vi "subSave_Dcimg2Bin.vi"(5 "Delete .dcimg? (T)":bool=TRUE, 7 "Text":string, 8 "Error in":errorcluster, 11 ".dcimg file name":path) -> (0 "Error out":errorcluster)   [LabVIEW 2015]
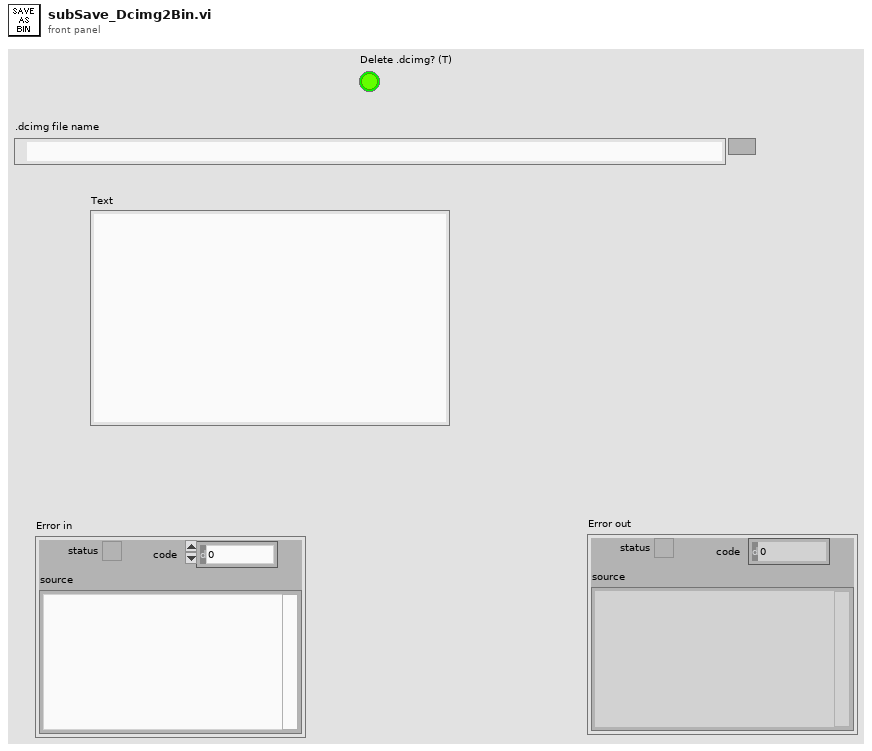
[diagram p1: front panel]
types:
  T1 = enum16{"open", "replace", "create", "open or create", "replace or create", "replace or create with confirmation"}
  T2 = enum16{"big-endian, network order", "native, host order", "little-endian"}
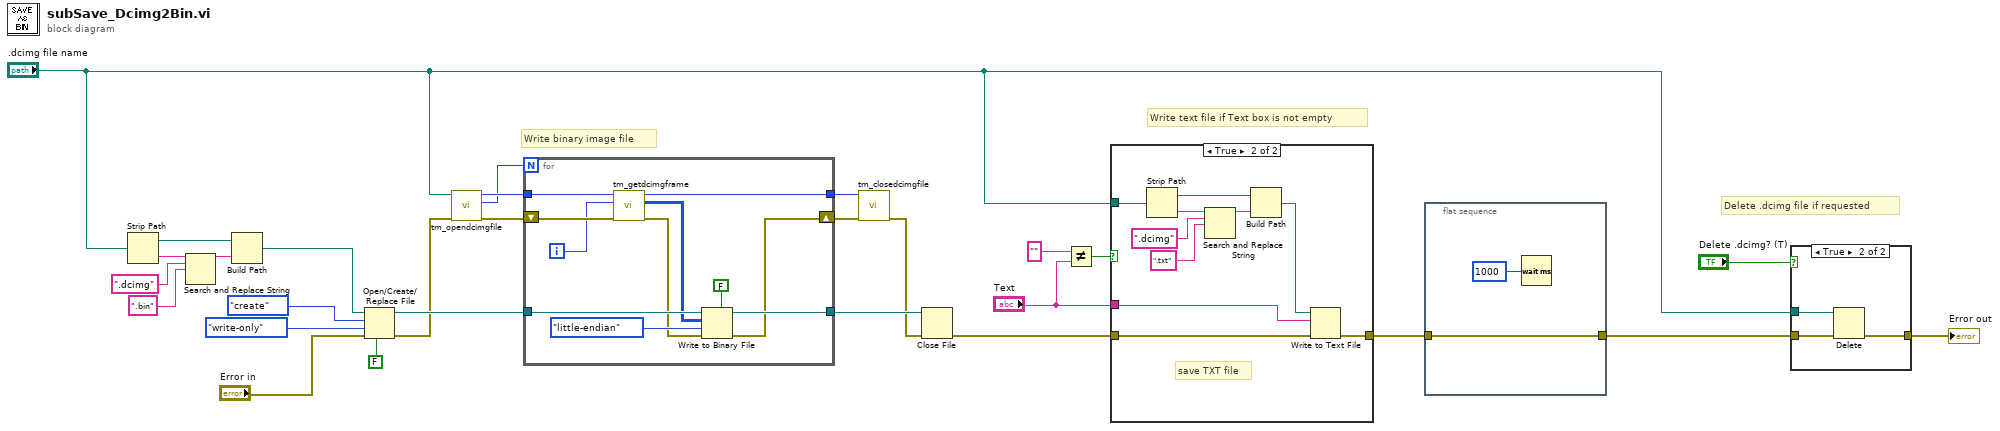
[diagram p0: block diagram]
diagram:
  # "Delete .dcimg file if requested"
  # "Write binary image file"
  # "Write text file if Text box is not empty"
  n1 = Strip Path(path=".dcimg file name") -> (stripped path=w18:path, name=w15:string)
  n2 = Search and Replace String(input string=w15, search string=".dcimg", replace string=".bin" ("replace string (\"\")")) -> (result string=w19:string)  [unwired: 5 in, 3 out]
  n3 = Build Path(base path=w18, name or relative path=w19) -> (appended path=w14:path)
  n4 = Open/Create/Replace File(file path (use dialog)=w14, error in="Error in", operation (0:open)=T1."create", access (0:read/write)=enum16{"read/write", "read-only", "write-only"}."write-only", disable buffering (F)=FALSE) -> (refnum out=w28:refnum<file>, error out=w12:errorcluster)  [unwired: 1 in, 1 out]
  n5 = call "tm_opendcimgfile.vi"("error in (no error)"=w12, "Path"=".dcimg file name") -> ("error out"=w26:errorcluster, "Total Frames"=w10:i32, "File Handle"=w27:u32)  [unwired: 7 in]
  n6 = for {
    N: w10 -> [_]
    shift-right: [w30] -> w25
    shift-left: w26 -> [w39]
    tunnel: w27 -> [w38]
    tunnel: [w37] -> w24
    tunnel: w28 -> [w35]
    tunnel: [w32] -> w23
    i -> [w31]
    n7 = call "tm_getdcimgframe.vi"("error in (no error)"=w39, "Frame Index"=w31, "File Handle in"=w38) -> ("error out"=w29:errorcluster, "Data"=w33:u16[][], "File Handle out"=w37:u32)  [unwired: 5 in, 1 out]
    n8 = Write to Binary File(file (use dialog)=w35, data=w33, error in=w29, 5:FALSE, 9:T2."little-endian" ("byte order (0:big-endian, network order)")) -> (refnum out=w32:refnum<file>, error out=w30:errorcluster)  [unwired: 1 in, 1 out]
  }
  n9 = call "tm_closedcimgfile.vi"("error in (no error)"=w25, "File Handle"=w24) -> ("error out"=w11:errorcluster)  [unwired: 9 in]
  n10 = Close File(refnum=w23, error in=w11) -> (error out=w6:errorcluster)  [unwired: 1 out]
  n11 = Not Equal?(x="", y="Text") -> (x != y?=w2:bool)
  n12 = case shown="True" w2 {
    tunnel: ".dcimg file name" -> [_ w44]
    tunnel: w6 -> [w40 w43]
    tunnel: [w40 w42] -> w5
    tunnel: "Text" -> [_ w41]
    frame False {
    }
    frame True {
      # "save TXT file"
      n13 = Strip Path(path=w44) -> (stripped path=w48:path, name=w45:string)
      n14 = Search and Replace String(input string=w45, search string=".dcimg", replace string=".txt" ("replace string (\"\")")) -> (result string=w49:string)  [unwired: 5 in, 3 out]
      n15 = Build Path(base path=w48, name or relative path=w49) -> (appended path=w50:path)
      n16 = Write to Text File(file (use dialog)=w50, text=w41, error in=w43) -> (error out=w42:errorcluster)  [unwired: 1 in, 2 out]
    }
  }
  n17 = flat-sequence {
    tunnel: w5 -> [w52]
    tunnel: [w52] -> w7
    frame #0 {
      n18 = Wait (ms)(milliseconds to wait=u32 1000) -> ()  [unwired: 1 out]
    }
  }
  n19 = case shown="True" "Delete .dcimg? (T)" {
    tunnel: w7 -> [w53 w56]
    tunnel: [w53 w55] -> w9
    tunnel: ".dcimg file name" -> [_ w54]
    frame False {
    }
    frame True {
      n20 = Delete(path (use dialog)=w54, error in=w56) -> (error out=w55:errorcluster)  [unwired: 3 in, 2 out]
    }
  }
  "Error out" <- w9
